vi "Validate Bundle File Path.vi"(8 "error in (no error)":errorcluster, 10 "Bundle File Path":path, 11 "Bundle Builder in":refnum<class "Bundle Builder.lvclass">) -> (0 "error out":errorcluster, 2 "Valid?":bool, 3 "Bundle Builder out":refnum<class "Bundle Builder.lvclass">)   [LabVIEW 2020, in "Bundle Builder.lvclass"]
uses:
  Bundle Builder.lvclass
  Bundle Builder.lvclass/Bundle Builder.ctl
  <vilib>/ErrorRing/Error Ring.xnode
  <vilib>/Utility/error.llb/Error Cluster From Error Code.vi
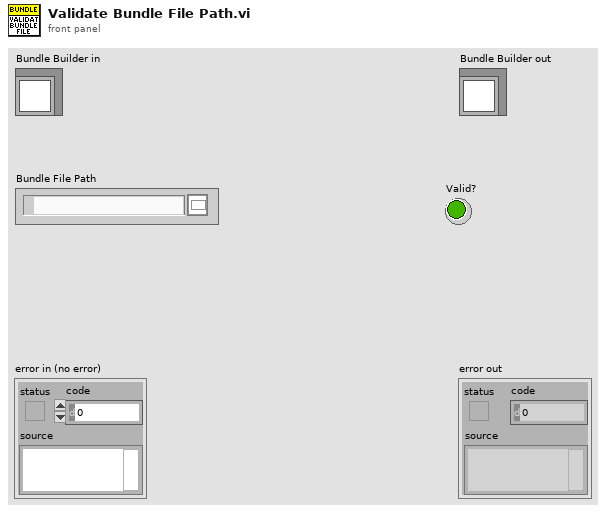
[diagram p1: front panel]
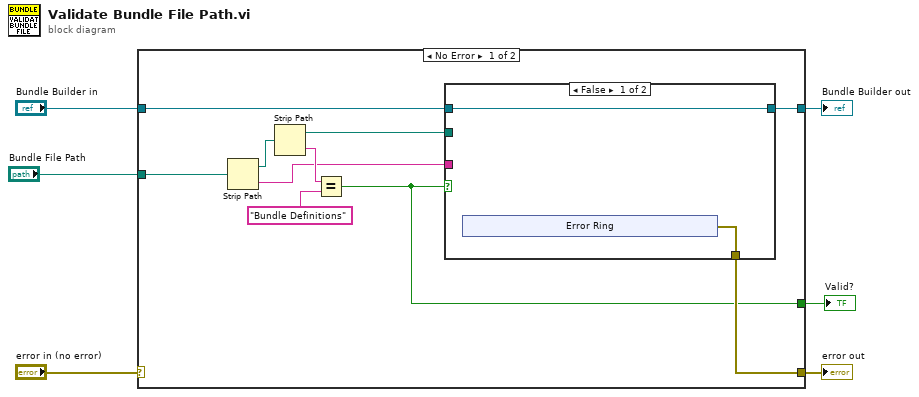
[diagram p0: block diagram]
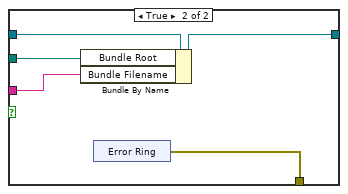
[diagram p2: hidden frame]
diagram:
  n1 = case shown="No Error" "error in (no error)" {
    selector: "error in (no error)" -> [_ w31]
    tunnel: [w8 w31] -> w5
    tunnel: [w11 w30] -> w3
    tunnel: "Bundle Builder in" -> [w16 w30]
    tunnel: "Bundle File Path" -> [w15 _]
    tunnel: [w7 _] -> w1
    frame No Error {
      n2 = Strip Path(path=w15) -> (stripped path=w14:path, name=w10:string)
      n3 = Strip Path(path=w14) -> (stripped path=w9:path, name=w13:string)
      n4 = Equal?(x=w13, y="Bundle Definitions") -> (x = y?=w7:bool)
      n5 = case shown="False" w7 {
        tunnel: w16 -> [w18 w28]
        tunnel: [w18 w27] -> w11
        tunnel: w10 -> [_ w26]
        tunnel: w9 -> [_ w25]
        tunnel: [w17 w24] -> w8
        frame False {
          n6 = xnode "Error Ring"() -> ("error out"=w17:errorcluster)
        }
        frame True {
          n7 = Bundle By Name(cluster=w28, "Bundle Root"=w25, "Bundle Filename"=w26) -> (w27:refnum<class "Bundle Builder.lvclass">)
          n8 = xnode "Error Ring"() -> ("error out"=w24:errorcluster)
        }
      }
    }
    frame Error {
    }
  }
  "error out" <- w5
  "Bundle Builder out" <- w3
  "Valid?" <- w1
